vi "test-filter-exec-MANUAL.vi"() -> ()   [LabVIEW 2019]
uses:
  <vilib>/Rock Robotics/WPI/ThirdParty/JAS_Junk/TrajLib/LINEAR_FILTER.ctl
  <vilib>/Rock Robotics/WPI/ThirdParty/JAS_Junk/TrajLib/LinearFilter_ResetToValue.vi
  <vilib>/Rock Robotics/WPI/ThirdParty/JAS_Junk/TrajLib/LinearFilter_Calculate.vi
  <vilib>/Rock Robotics/WPI/ThirdParty/JAS_Junk/TrajLib/LinearFilter_MovingAverage.vi
  <vilib>/Rock Robotics/WPI/ThirdParty/JAS_Junk/TrajLib/LinearFilter_LowPassBW1.vi
  <vilib>/Rock Robotics/WPI/ThirdParty/JAS_Junk/TrajLib/LinearFilter_LowPassBW2.vi
  <vilib>/Rock Robotics/WPI/ThirdParty/JAS_Junk/TrajLib/LinearFilter_HighPassBW1.vi
  <vilib>/Rock Robotics/WPI/ThirdParty/JAS_Junk/TrajLib/LinearFilter_HighPassBW2.vi
  <vilib>/Rock Robotics/WPI/ThirdParty/JAS_Junk/TrajLib/Util_LibraryGlobals.vi
  <vilib>/Rock Robotics/WPI/ThirdParty/JAS_Junk/TrajLib/Trajectory_Library.lvlib
panel:
  out "LibUsage_ProfiledPID":i32 format="%20.0f"
  out "LibUsage_PIDController":i32 format="%20.0f"
  out "LibUsage_Odometry":i32 format="%20.0f"
  out "LibUsage_LinearFIlter":i32 format="%20.0f"
  out "LibUsage_TrapezoidProfile":i32 format="%20.0f"
  out "LibUsage_Kinematics":i32 format="%20.0f"
  in  "Random noise amplitude":bool
  out "time diff":u32
  out "High BW2":T1 {"Outputs" format="%13.5g"; "Inputs" format="%13.5g"; "OutputGains" format="%13.5g"; "InputGains" format="%13.5g"}
  in  "noise Offset - millliseconds":dbl format="%14.5g"
  out "Cutoff Freq":dbl format="%14.5g"
  out "High BW1":T1 {"Outputs" format="%13.5g"; "Inputs" format="%13.5g"; "OutputGains" format="%13.5g"; "InputGains" format="%13.5g"}
  out "High Pass":T1 {"Outputs" format="%13.5g"; "Inputs" format="%13.5g"; "OutputGains" format="%13.5g"; "InputGains" format="%13.5g"}
  out "mov Avg":T1 {"Outputs" format="%13.5g"; "Inputs" format="%13.5g"; "OutputGains" format="%13.5g"; "InputGains" format="%13.5g"}
  in  "MovAvgSamp":i32 format="%14.5g"
  out "BW 2":T1 {"Outputs" format="%13.5g"; "Inputs" format="%13.5g"; "OutputGains" format="%13.5g"; "InputGains" format="%13.5g"}
  out "BW 1":T1 {"Outputs" format="%13.5g"; "Inputs" format="%13.5g"; "OutputGains" format="%13.5g"; "InputGains" format="%13.5g"}
  out "Single pole":T1 {"Outputs" format="%13.5g"; "Inputs" format="%13.5g"; "OutputGains" format="%13.5g"; "InputGains" format="%13.5g"}
  in  "Noise Amplitude":dbl(slide)=1.0 scale=0.0..10.0
  in  "TimeConstant":dbl format="%14.5g"
  in  "Noise Frequency":dbl(slide)=0.2 min=0.1 max=1000.0 step=0.5 scale=0.1..1000.0 scale format="%14.5g"
  out "Waveform Chart":T2(graph)
  in  "Primary Frequency":dbl(slide)=0.2 min=0.1 max=1000.0 step=0.5 scale=0.1..10.0 scale format="%14.5g"
  in  "Amplitude":dbl(slide)=1.0 scale=0.0..10.0
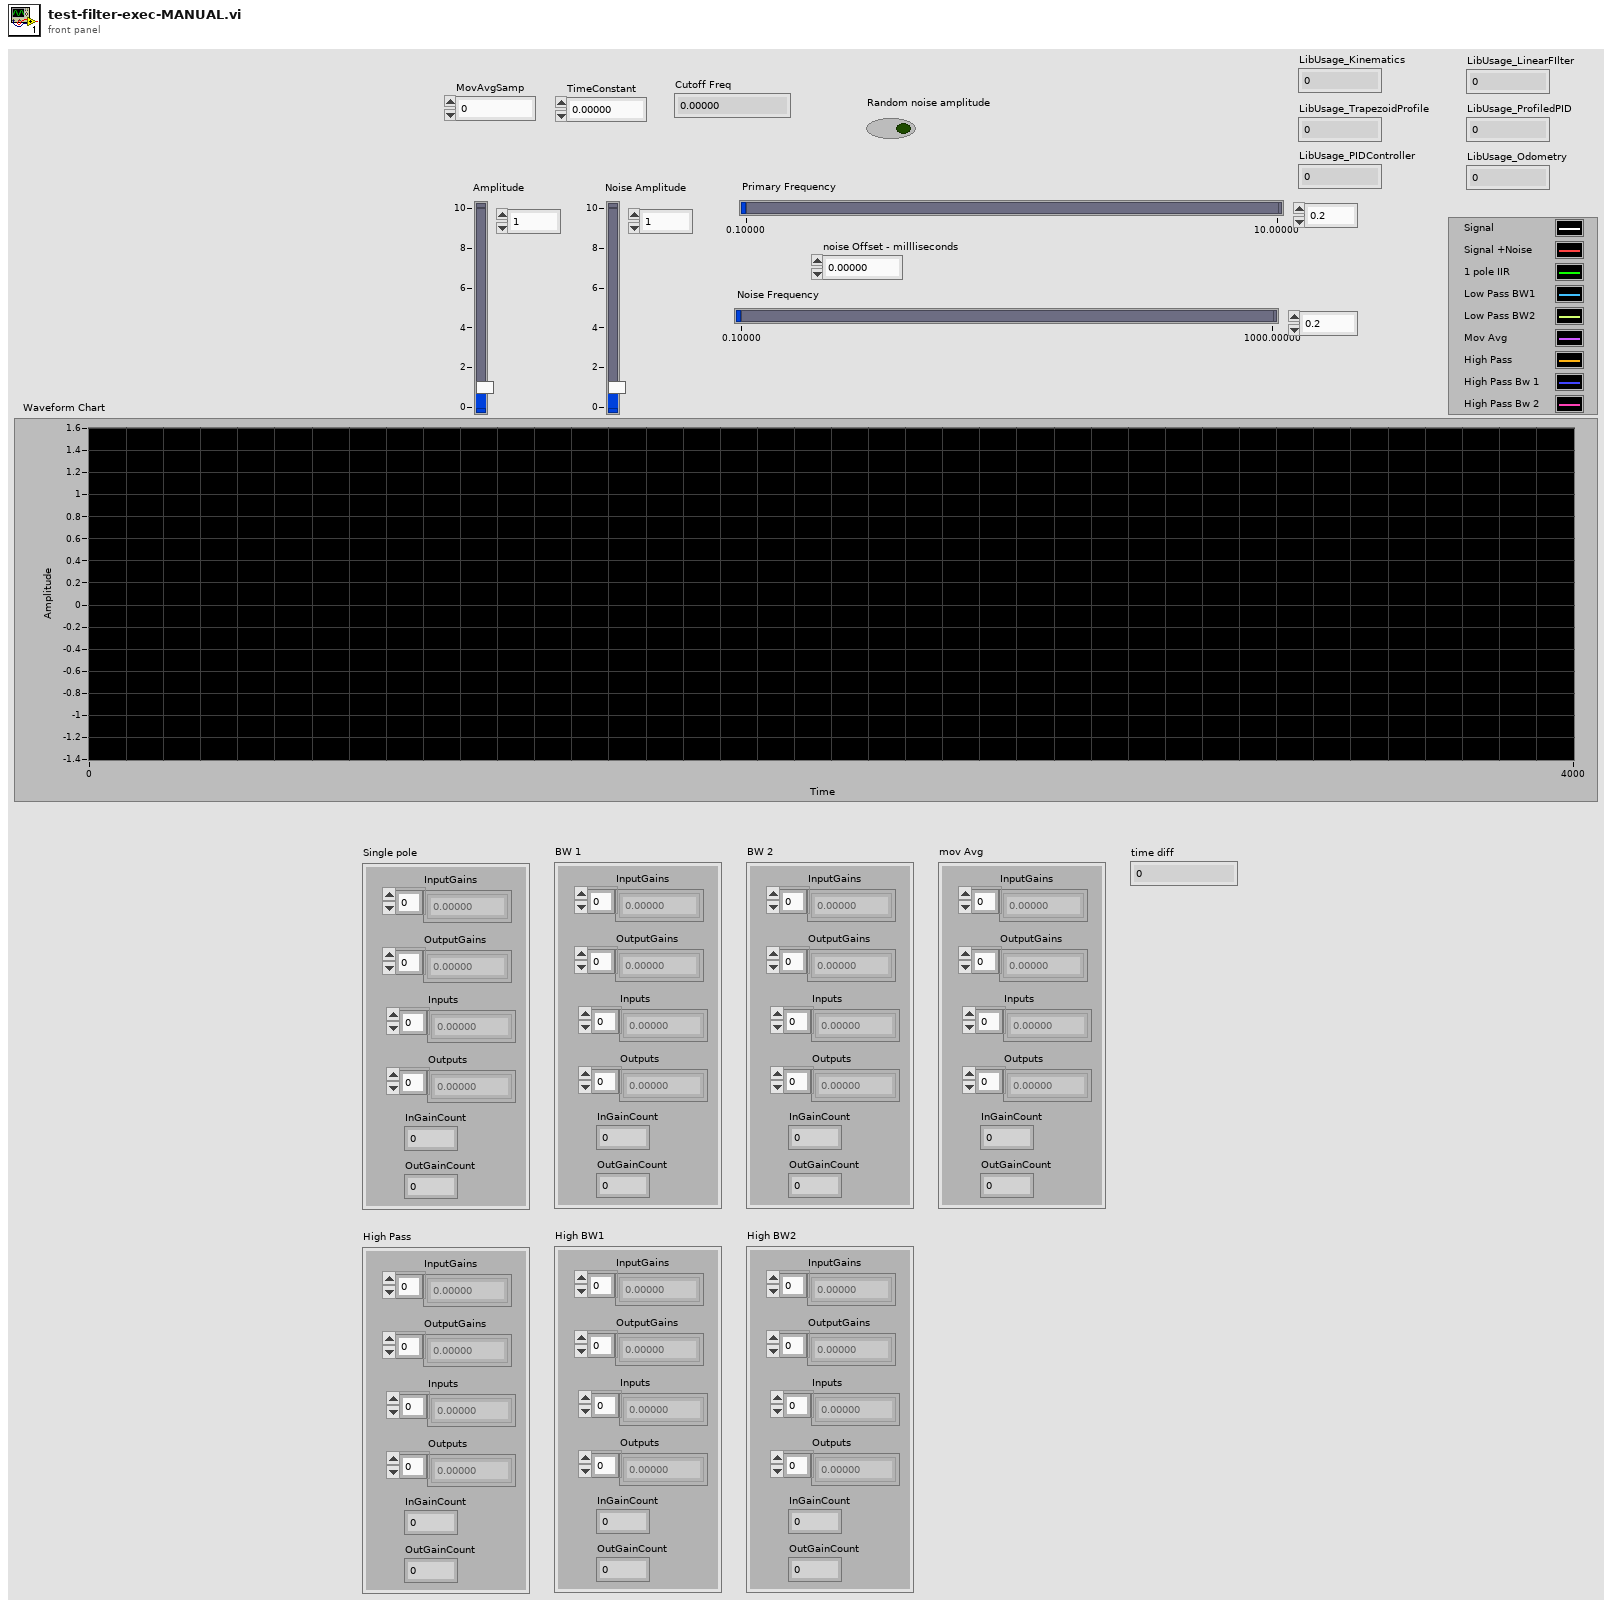
[diagram p1: front panel]
types:
  T1 = typedef "Trajectory_Library.lvlib/LINEAR_FILTER.ctl" = cluster{"InputGains":dbl[], "OutputGains":dbl[], "Inputs":dbl[], "Outputs":dbl[], "InGainCount":i32, "OutGainCount":i32}
  T2 = cluster{dbl, dbl, "Output":dbl, "Output":dbl, "Output":dbl, "Output":dbl, "Output":dbl, "Output":dbl, "Output":dbl}
  T3 = enum16{"Moving Average", "Low Pass 1st Order Butterworth", "Low Pass 2nd Order Butterworth", "High Pass 1st Order Butterworth", "High Pass 2nd Order Butterworth"}
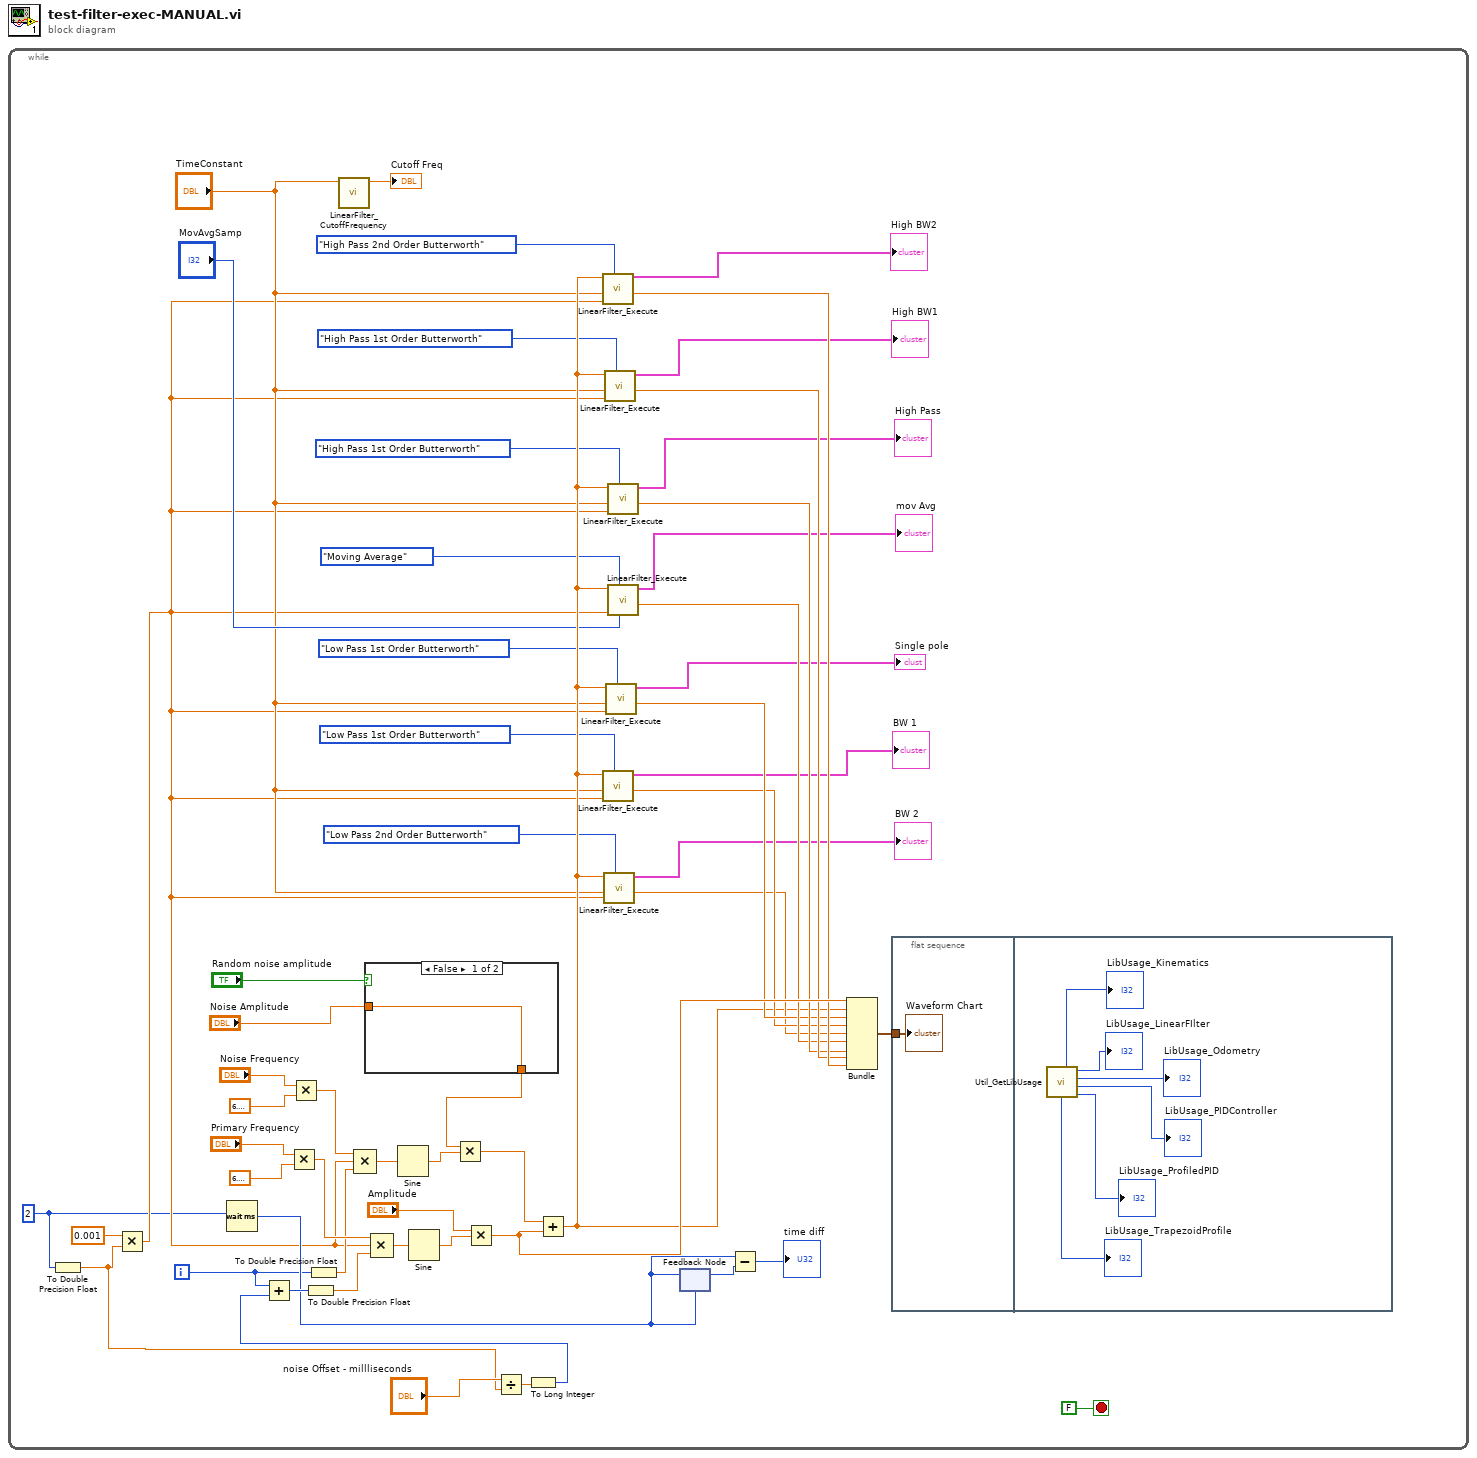
[diagram p0: block diagram]
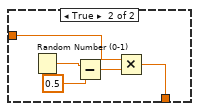
[diagram p2: hidden frame]
diagram:
  n1 = while {
    i -> [w34]
    stop <- FALSE stop-if-true
    w2 = u32 2 ("milliseconds to wait")
    n2 = To Double Precision Float(number=w2) -> (double precision float=w3:dbl)
    n3 = Multiply(x=0.001 ("value"), y=w3) -> (x*y=w4:dbl)
    n4 = Wait (ms)(milliseconds to wait=w2) -> (millisecond timer value=w36:u32)
    n5 = Multiply(x="Primary Frequency", y=6.283185307179586) -> (x*y=w46:dbl)
    n6 = Multiply(x="Noise Frequency", y=6.283185307179586) -> (x*y=w47:dbl)
    n7 = To Double Precision Float(number=w34) -> (double precision float=w45:dbl)
    n8 = call <vilib>:"LinearFilter_CutoffFrequency.vi"("TimeConstant"="TimeConstant") -> ("Cutoff Freq"=→"Cutoff Freq":dbl)  [unwired: 10 in]
    n9 = Compound Arithmetic op=MULTIPLY(w47, w4, w45) -> (w49:dbl)
    n10 = case shown="False" "Random noise amplitude" {
      tunnel: "Noise Amplitude" -> [w65 w67]
      tunnel: [w65 w66] -> w31
      frame False {
      }
      frame True {
        n11 = Random Number (0-1)() -> (number: 0 to 1=w70:dbl)
        n12 = Subtract(x=w70, y=0.5) -> (x-y=w68:dbl)
        n13 = Multiply(x=w67, y=w68) -> (x*y=w66:dbl)
      }
    }
    n14 = Sine(x=w49) -> (sin(x)=w48:dbl)
    n15 = Multiply(x=w31, y=w48) -> (x*y=w44:dbl)
    n16 = Divide(x="noise Offset - millliseconds", y=w3) -> (x/y=w40:dbl)
    n17 = To Long Integer(number=w40) -> (32bit integer=w38:i32)
    n18 = Add(x=w34, y=w38) -> (x+y=w42:i32)
    n19 = To Double Precision Float(number=w42) -> (double precision float=w41:dbl)
    n20 = Compound Arithmetic op=MULTIPLY(w46, w4, w41) -> (w57:dbl)
    n21 = Sine(x=w57) -> (sin(x)=w56:dbl)
    n22 = Multiply(x="Amplitude", y=w56) -> (x*y=w43:dbl)
    n23 = Add(x=w44, y=w43) -> (x+y=w23:dbl)
    n24 = call <vilib>:"LinearFilter_Execute.vi"("Filter Type"=T3."High Pass 2nd Order Butterworth", "SamplePeriod"=w4, "TimeConstant"="TimeConstant", "Input"=w23) -> ("Output"=w30:dbl, "Out LINEAR_FILTER"=→"High BW2":T1)  [unwired: 6 in]
    n25 = call <vilib>:"LinearFilter_Execute.vi"("Filter Type"=T3."Low Pass 1st Order Butterworth", "SamplePeriod"=w4, "TimeConstant"="TimeConstant", "Input"=w23) -> ("Output"=w25:dbl, "Out LINEAR_FILTER"=→"BW 1":T1)  [unwired: 6 in]
    n26 = call <vilib>:"LinearFilter_Execute.vi"("Filter Type"=T3."Low Pass 2nd Order Butterworth", "SamplePeriod"=w4, "TimeConstant"="TimeConstant", "Input"=w23) -> ("Output"=w24:dbl, "Out LINEAR_FILTER"=→"BW 2":T1)  [unwired: 6 in]
    n27 = call <vilib>:"LinearFilter_Execute.vi"("Filter Type"=T3."High Pass 1st Order Butterworth", "SamplePeriod"=w4, "TimeConstant"="TimeConstant", "Input"=w23) -> ("Output"=w29:dbl, "Out LINEAR_FILTER"=→"High BW1":T1)  [unwired: 6 in]
    n28 = call <vilib>:"LinearFilter_Execute.vi"("Filter Type"=T3."Low Pass 1st Order Butterworth", "SamplePeriod"=w4, "TimeConstant"="TimeConstant", "Input"=w23) -> ("Output"=w26:dbl, "Out LINEAR_FILTER"=→"Single pole":T1)  [unwired: 6 in]
    n29 = call <vilib>:"LinearFilter_Execute.vi"("Filter Type"=T3."High Pass 1st Order Butterworth", "SamplePeriod"=w4, "TimeConstant"="TimeConstant", "Input"=w23) -> ("Output"=w28:dbl, "Out LINEAR_FILTER"=→"High Pass":T1)  [unwired: 6 in]
    n30 = call <vilib>:"LinearFilter_Execute.vi"("Samples"="MovAvgSamp", "Filter Type"=T3."Moving Average", "SamplePeriod"=w4, "Input"=w23) -> ("Output"=w27:dbl, "Out LINEAR_FILTER"=→"mov Avg":T1)  [unwired: 6 in]
    n31 = feedback-in #1(w36) -> ()
    n32 = feedback #1(w36) -> (w37:u32)
    n33 = Subtract(x=w36, y=w37) -> (x-y=→"time diff":u32)
    n34 = Bundle(w43, w23, "Output"=w26, "Output"=w25, "Output"=w24, "Output"=w27, "Output"=w28, "Output"=w29, "Output"=w30) -> (w54:T2)  [unwired: 1 in]
    n35 = flat-sequence {
      tunnel: w54 -> [w58]
      frame #0 {
        "Waveform Chart" <- w58
      }
      frame #1 {
        n36 = call <vilib>:"Util_GetLibUsage.vi"() -> ("LibUsage_ProfiledPID"=→"LibUsage_ProfiledPID":i32, "LibUsage_PIDController"=→"LibUsage_PIDController":i32, "LibUsage_Odometry"=→"LibUsage_Odometry":i32, "LibUsage_LinearFIlter"=→"LibUsage_LinearFIlter":i32, "LibUsage_TrapezoidProfile"=→"LibUsage_TrapezoidProfile":i32, "LibUsage_Kinematics"=→"LibUsage_Kinematics":i32)  [unwired: 6 in]
      }
    }
  }
